vi "waitToStopServerProcess.vi"(8 "error in (no error)":errorcluster, 11 "tcpServer in":refnum<class "TcpServer.lvclass">) -> (0 "error out":errorcluster, 1 "timed out?":bool, 2 "stopProcess":bool, 3 "tcpServer out":refnum<class "TcpServer.lvclass">)   [LabVIEW 2018, in "TcpServer.lvclass"]
doc: "Wait to stop a process inside runServer.vi. This is a non-block call function.\n\nNOTE: put this VI in preallocated reentrant clone execution."
uses:
  TcpServer.lvclass
  TcpServer.lvclass/TcpServer.ctl
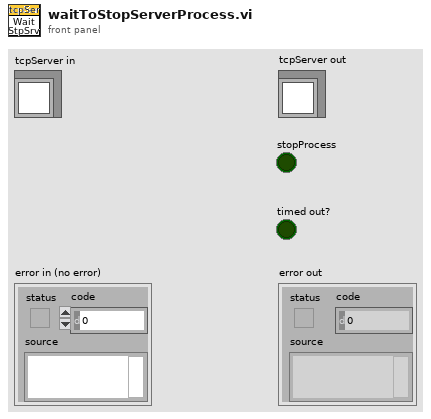
[diagram p1: front panel]
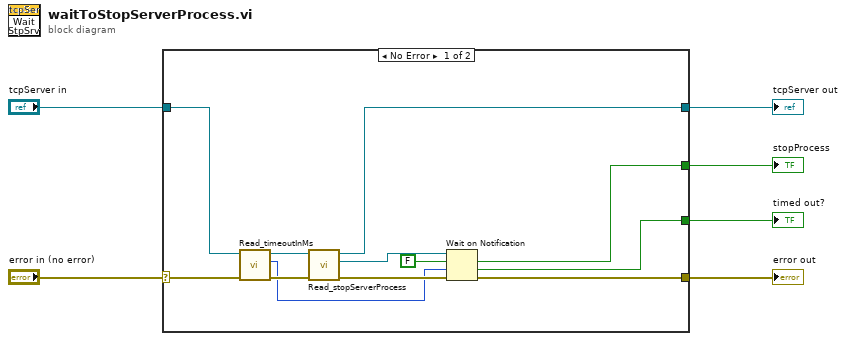
[diagram p0: block diagram]
diagram:
  n1 = case shown="No Error" "error in (no error)" {
    selector: "error in (no error)" -> [w11 w19]
    tunnel: [w17 w19] -> w5
    tunnel: "tcpServer in" -> [w8 w20]
    tunnel: [w14 _] -> w3
    tunnel: [w13 _] -> w2
    tunnel: [w12 w20] -> w1
    frame No Error {
      n2 = call "Read_timeoutInMs.vi"("error in (no error)"=w11, "TcpServer in"=w8) -> ("error out"=w10:errorcluster, "timeoutInMs"=w7:i32, "TcpServer out"=w9:refnum<class "TcpServer.lvclass">)  [unwired: 7 in]
      n3 = call-dynamic "Read_stopServerProcess.vi"("error in (no error)"=w10, "TcpServer in"=w9) -> ("error out"=w18:errorcluster, "stopServerProcessNotifier"=w16:refnum<notifier>, "TcpServer out"=w12:refnum<class "TcpServer.lvclass">)  [unwired: 7 in]
      n4 = Wait on Notification(notifier=w16, ignore previous (F)=FALSE, timeout in ms (-1)=w7, error in (no error)=w18) -> (notification=w14:bool, timed out?=w13:bool, error out=w17:errorcluster)  [unwired: 1 out]
    }
    frame Error {
    }
  }
  "error out" <- w5
  "tcpServer out" <- w1
  "stopProcess" <- w3
  "timed out?" <- w2
